vi "GetStringInfo.vi"(0 "reference in":refnum<class "StateNode.lvclass">, 5 "error in (no error)":errorcluster) -> (14 "reference out":refnum<class "StateNode.lvclass">, 15 "State":string, 16 "Action":string, 19 "error out":errorcluster)   [LabVIEW 2016, in "StateNode.lvclass"]
uses:
  <resource>/Framework/Providers/Open_GDS/UML/StateNode_class/StateNode.lvclass
  <resource>/Framework/Providers/Open_GDS/UML/MultiLineString_class/MultiLineString.lvclass
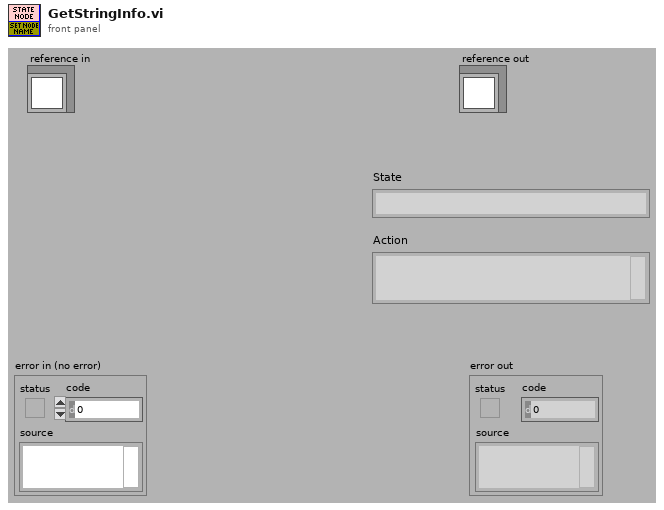
[diagram p1: front panel]
types:
  T1 = typedef "StateNode.lvclass/ObjectAttributes.ctl" = cluster{"state":refnum<class "MultiLineString.lvclass">, "action":refnum<class "MultiLineString.lvclass">, "DEFAULT_WIDTH":i32, "DEFAULT_HEIGHT":i32}
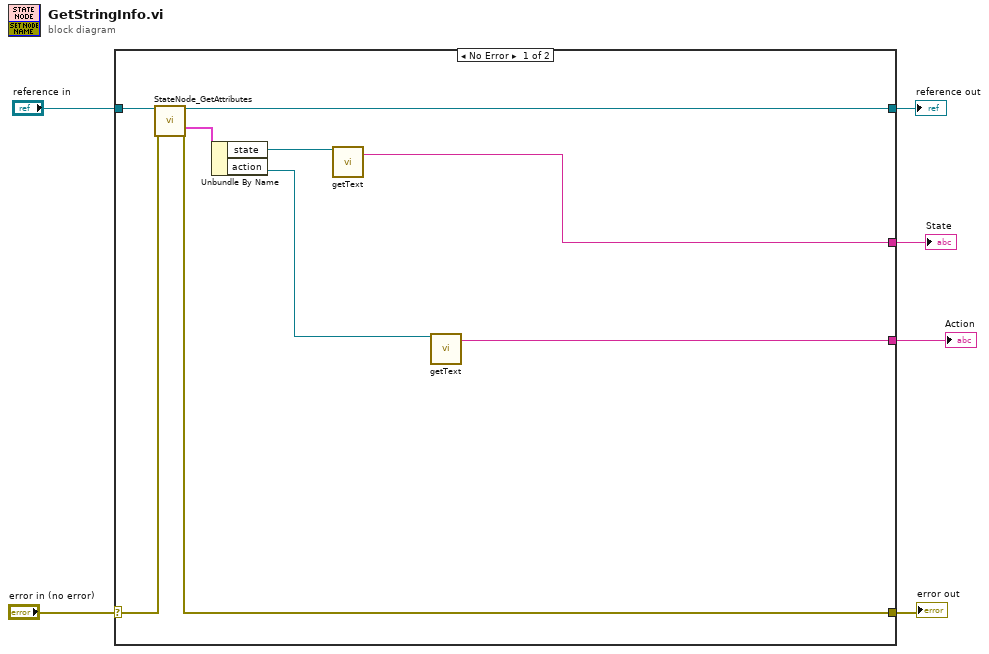
[diagram p0: block diagram]
diagram:
  n1 = case shown="No Error" "error in (no error)" {
    selector: "error in (no error)" -> [w15 w17]
    tunnel: [w14 w17] -> w5
    tunnel: [w12 w16] -> w3
    tunnel: "reference in" -> [w13 w16]
    tunnel: [w10 _] -> w2
    tunnel: [w8 _] -> w1
    frame No Error {
      n2 = call <resource>:"StateNode_GetAttributes.vi"("reference in"=w13, "error in (no error)"=w15) -> ("reference out"=w12:refnum<class "StateNode.lvclass">, "Data"=w7:T1, "error out"=w14:errorcluster)  [unwired: 14 in, 1 out]
      n3 = Unbundle By Name(w7) -> ("state"=w11:refnum<class "MultiLineString.lvclass">, "action"=w9:refnum<class "MultiLineString.lvclass">)
      n4 = call-dynamic "getText.vi"("reference"=w11) -> ("text"=w10:string)  [unwired: 16 in, 2 out]
      n5 = call-dynamic "getText.vi"("reference"=w9) -> ("text"=w8:string)  [unwired: 16 in, 2 out]
    }
    frame Error {
    }
  }
  "error out" <- w5
  "reference out" <- w3
  "State" <- w2
  "Action" <- w1
